vi "KeithleMatrixResistance.vi"() -> ()   [LabVIEW 2014]
uses:
  <vilib>/Utility/file.llb/Write To Spreadsheet File (DBL).vi
panel:
  out "Resistance":dbl
  out "Array":bool[][](array[boolean])
  in  "GPIB Address":string="12"
  out "String":string
  in  "Set values for testing contacts":bool
  out "Output Current (A)":dbl
  out "Output Voltage (V)":dbl
  out "Compliance limit (V)":dbl
  out "Current Range":u16(ring) items=["100 nA", "1 uA", "10 uA", "100 uA", "1 mA", "10 mA", "100 mA", "1 A"]
  out "Voltage Range":u16(ring) items=["200 mV", "2 V", "20 V", "200 V"]
  out "Current (sourse)":dbl
  out "Voltage (sourse)":dbl
  out "ComplianceIndicator":bool
  out "Compliance limit (A)":dbl
  out "Source Function":u16(ring)=1 items=["Current Source", "Voltage Source"]
  out "Sence Mode":u16(ring) items=["2-wire", "4-wire"]
  in  "ON/OFF channel":bool
  out "ON/OFF indicator":bool
  in  "error in (no error)":errorcluster
  out "error out":errorcluster
  # "Channel\nB"
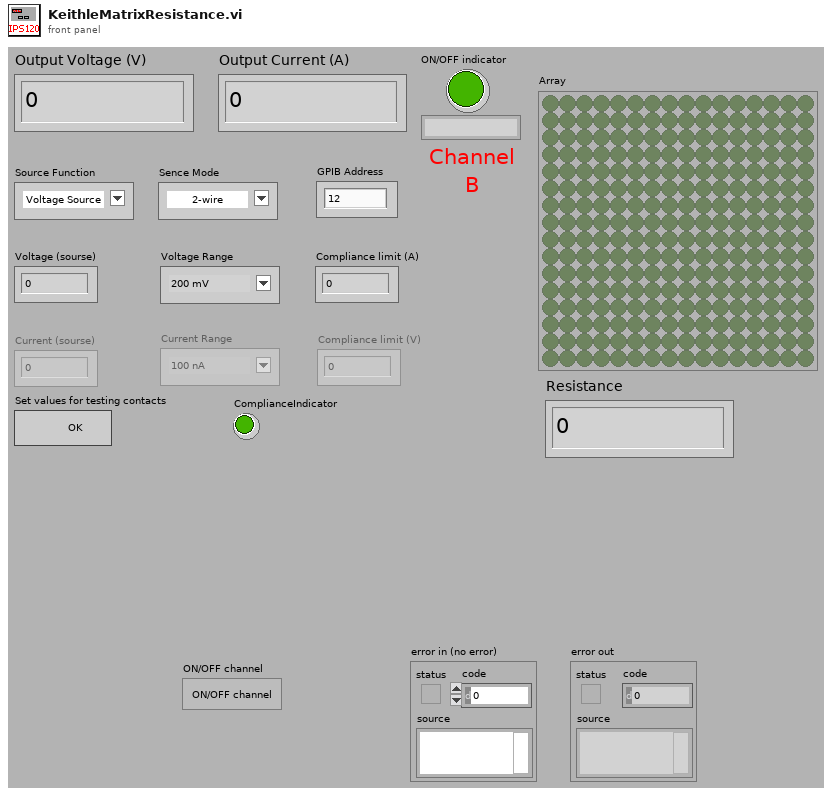
[diagram p1: front panel]
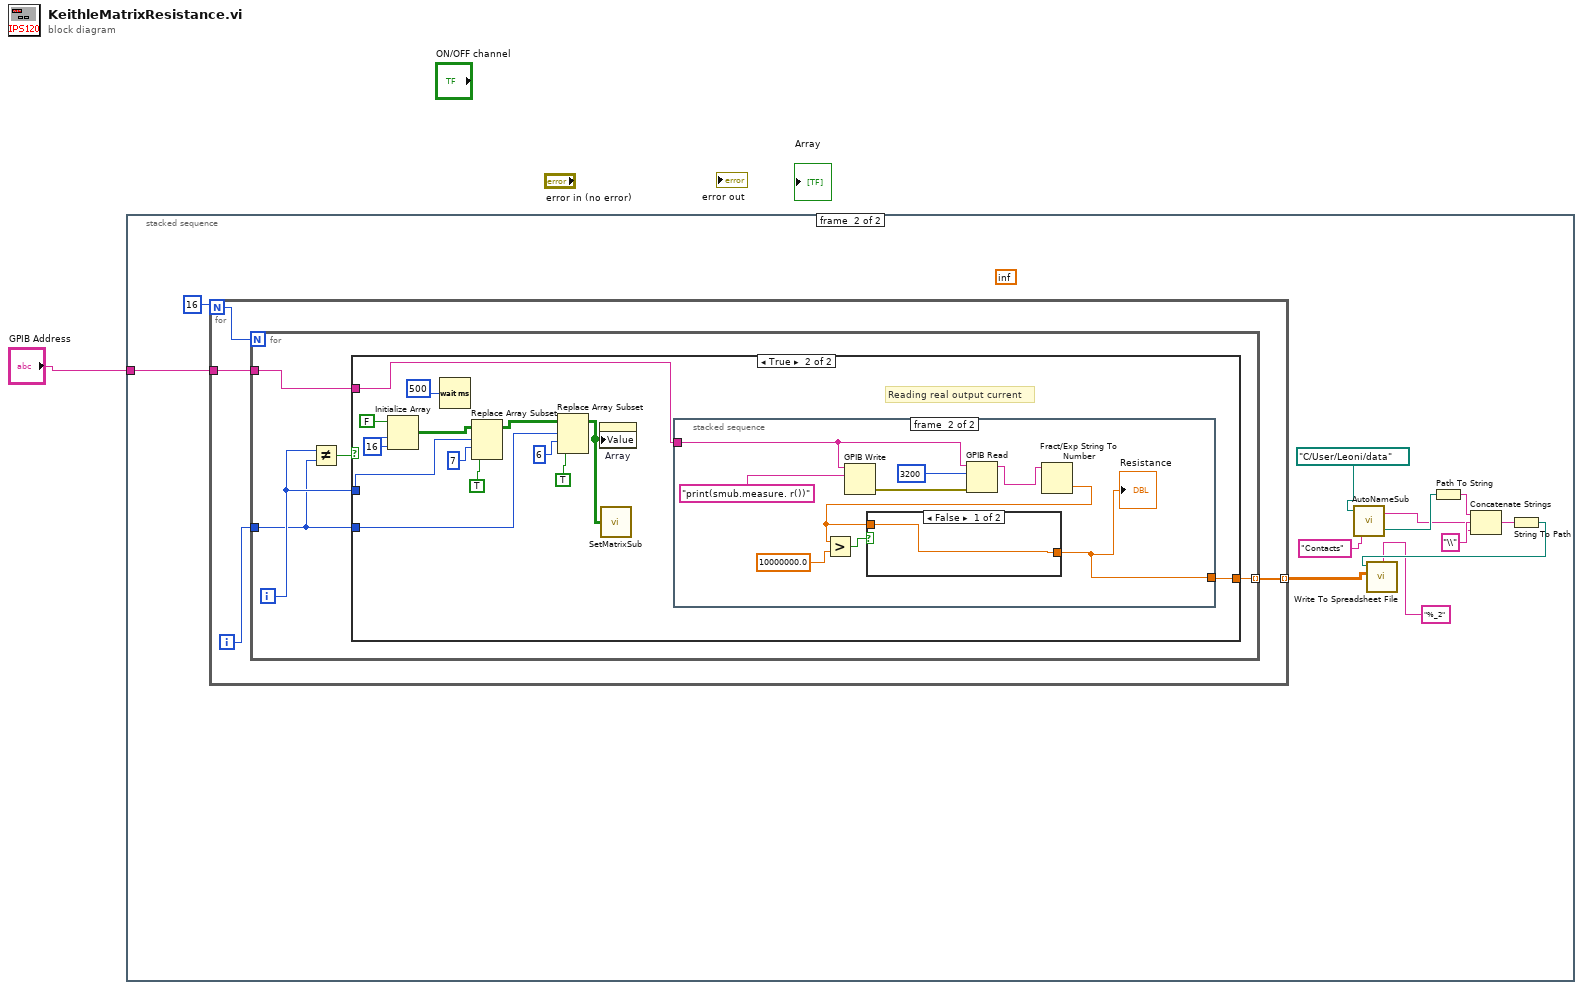
[diagram p0: block diagram]
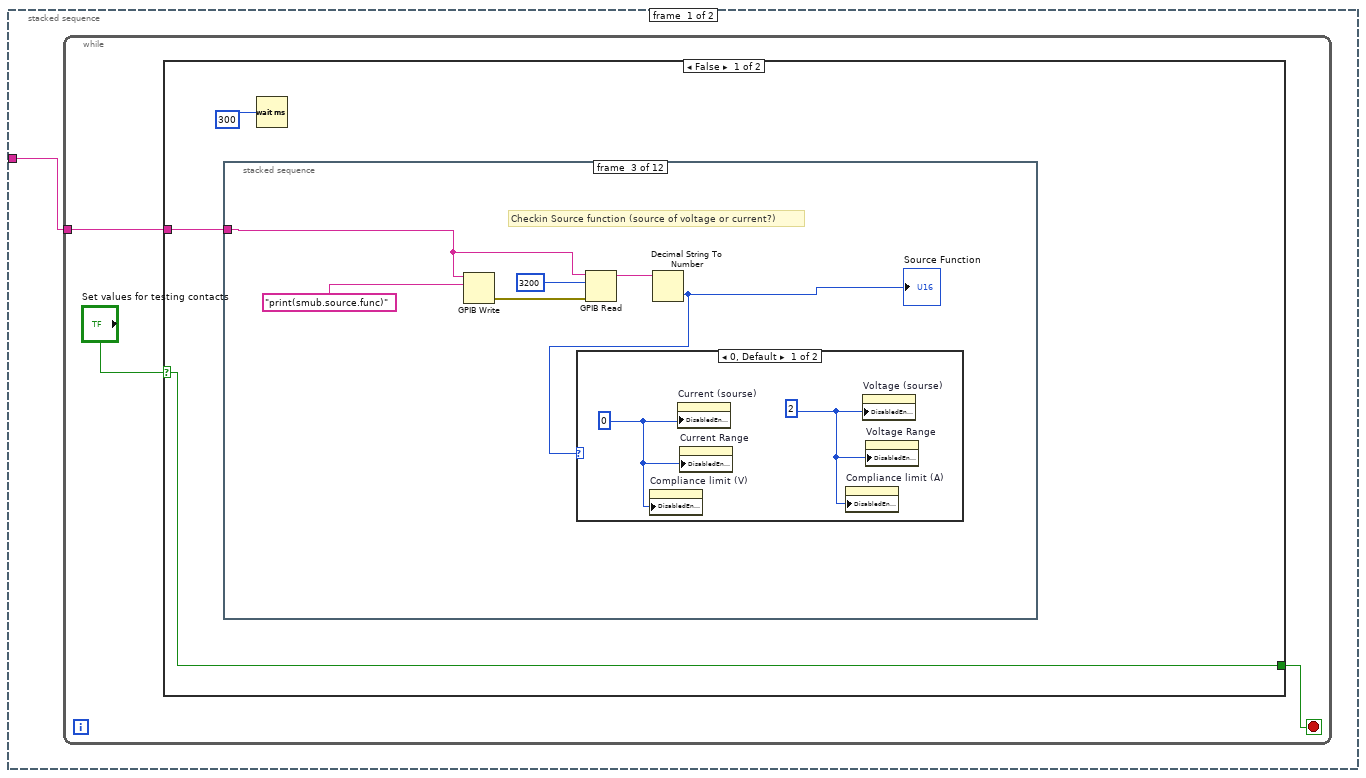
[diagram p2: hidden frame]
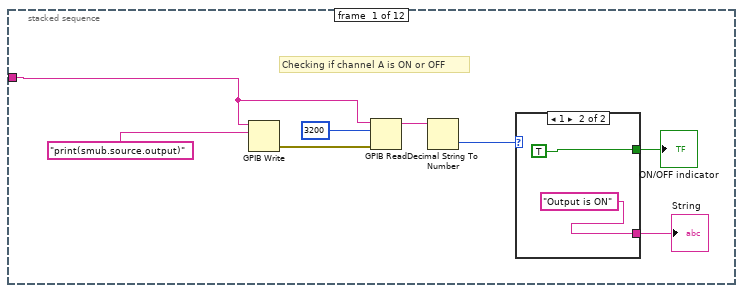
[diagram p3: hidden frame]
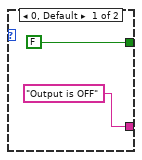
[diagram p4: hidden frame]
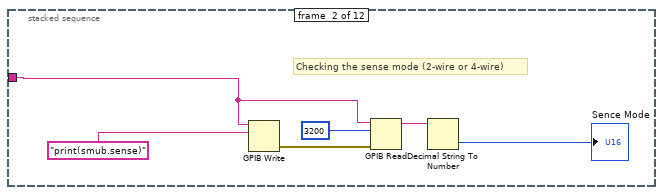
[diagram p5: hidden frame]
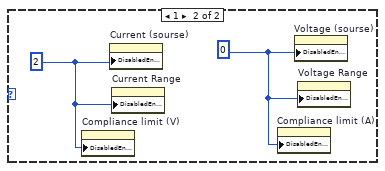
[diagram p6: hidden frame]
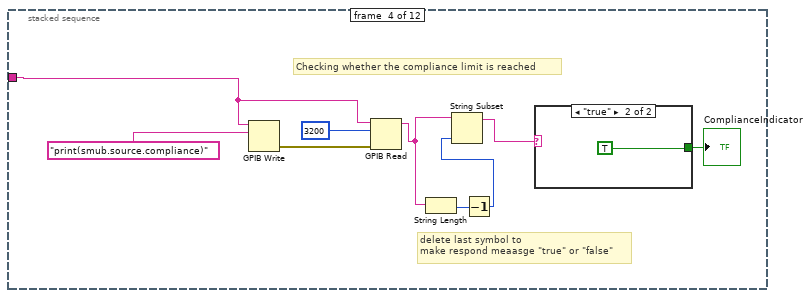
[diagram p7: hidden frame]
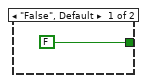
[diagram p8: hidden frame]
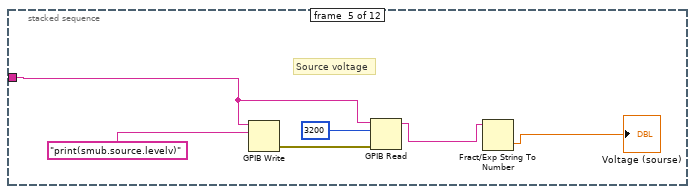
[diagram p9: hidden frame]
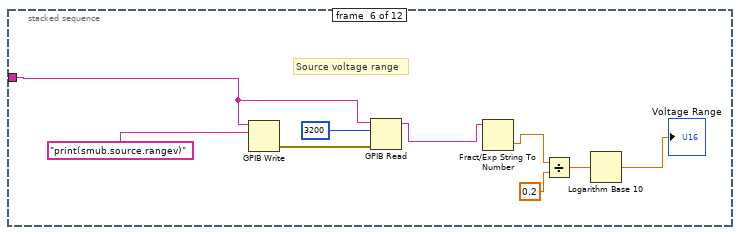
[diagram p10: hidden frame]
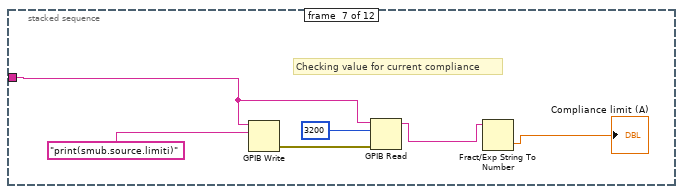
[diagram p11: hidden frame]
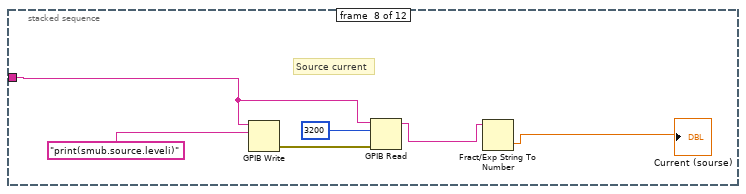
[diagram p12: hidden frame]
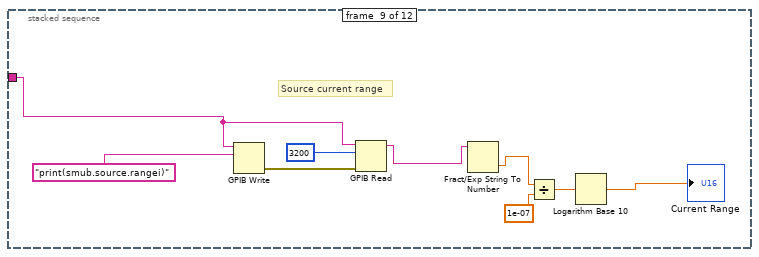
[diagram p13: hidden frame]
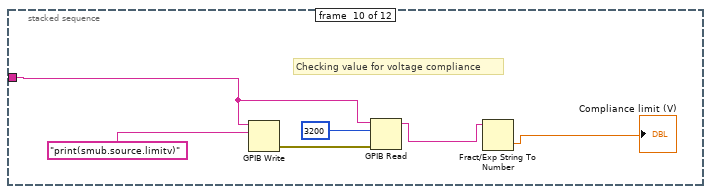
[diagram p14: hidden frame]
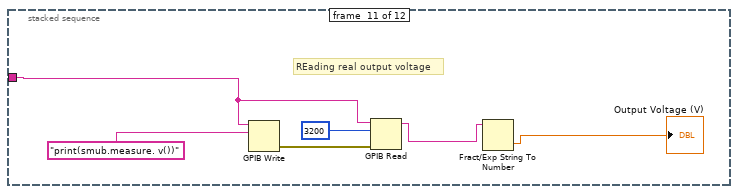
[diagram p15: hidden frame]
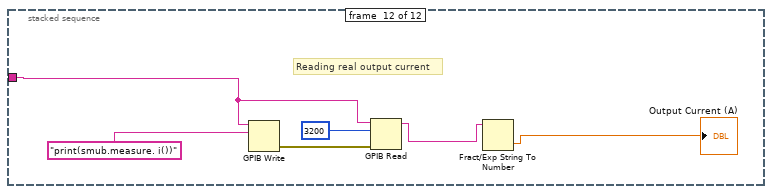
[diagram p16: hidden frame]
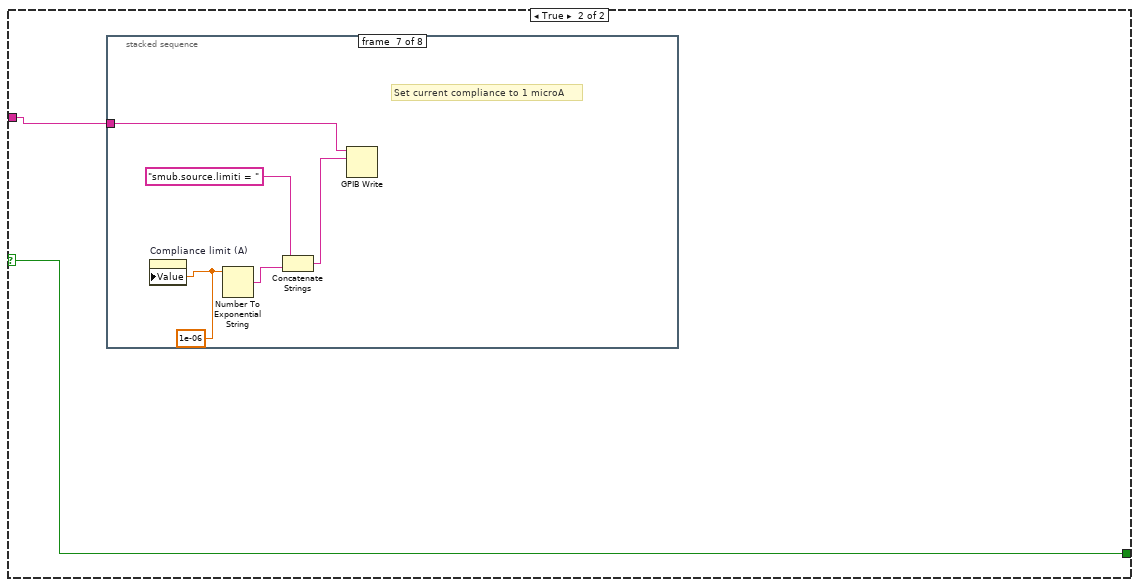
[diagram p17: hidden frame]
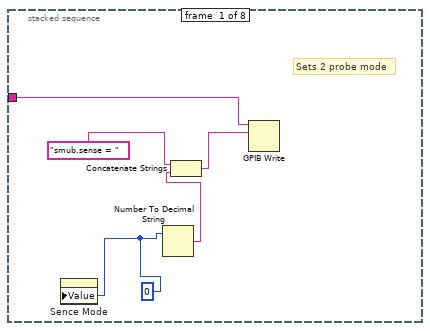
[diagram p18: hidden frame]
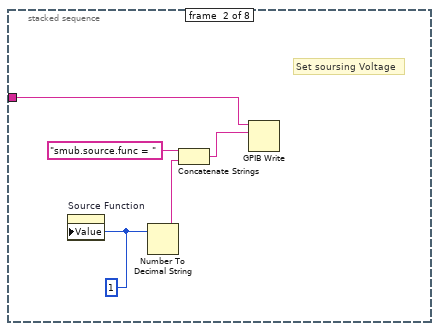
[diagram p19: hidden frame]
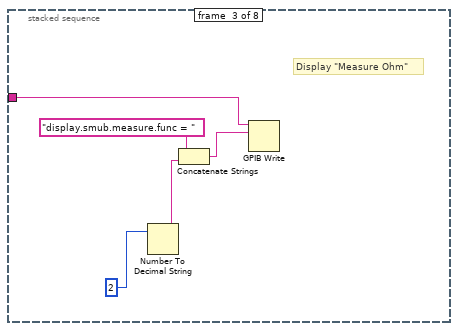
[diagram p20: hidden frame]
diagram:
  n1 = stacked-sequence {
    tunnel: "GPIB Address" -> [w2 w153]
    frame #0 {
      n2 = while {
        tunnel: w2 -> [w3]
        stop <- w4 stop-if-true
        n3 = case shown="False" "Set values for testing contacts" {
          selector: "Set values for testing contacts" -> [w7 w102]
          tunnel: w3 -> [w8 w103]
          tunnel: [w7 w102] -> w4
          frame False {
            n4 = stacked-sequence {
              tunnel: w8 -> [w9 w21 w27 w37 w48 w54 w63 w69 w75 w84 w90 w96]
              frame #0 {
                # "Checking if channel A is ON or OFF"
                n5 = GPIB Write(0:w9, 1:"print(smub.source.output)") -> (6:w16:errorcluster)  [unwired: 3 in, 1 out]
                n6 = GPIB Read(0:w9, 1:3200, 3:w16) -> (5:w13:string)  [unwired: 2 in, 2 out]
                n7 = Decimal String To Number(string=w13) -> (number=w12:i32)  [unwired: 2 in, 1 out]
                n8 = case shown="1" w12 {
                  tunnel: [FALSE TRUE] -> w11
                  tunnel: ["Output is OFF" "Output is ON"] -> w10
                  frame 0, Default {
                  }
                  frame 1 {
                  }
                }
                "ON/OFF indicator" <- w11
                "String" <- w10
              }
              frame #1 {
                # "Checking the sense mode (2-wire or 4-wire)"
                n9 = GPIB Write(0:w21, 1:"print(smub.sense)") -> (6:w26:errorcluster)  [unwired: 3 in, 1 out]
                n10 = GPIB Read(0:w21, 1:3200, 3:w26) -> (5:w23:string)  [unwired: 2 in, 2 out]
                n11 = Decimal String To Number(string=w23) -> (number=→"Sence Mode":i32)  [unwired: 2 in, 1 out]
              }
              frame #2 {
                # "Checkin Source function (source of voltage or current?)"
                n12 = GPIB Write(0:w27, 1:"print(smub.source.func)") -> (6:w32:errorcluster)  [unwired: 3 in, 1 out]
                n13 = GPIB Read(0:w27, 1:3200, 3:w32) -> (5:w29:string)  [unwired: 2 in, 2 out]
                n14 = Decimal String To Number(string=w29) -> (number=w28:i32)  [unwired: 2 in, 1 out]
                "Source Function" <- w28
                n15 = case shown="0, Default" w28 {
                  frame 0, Default {
                    w33 = 2
                    w34 = 0
                    n16 = property on="Compliance limit (V)" class="DigNum (strict)"("DisabledEnum"=w34) -> ()  [unwired: 2 in, 2 out]
                    n17 = property on="Current (sourse)" class="DigNum (strict)"("DisabledEnum"=w34) -> ()  [unwired: 2 in, 2 out]
                    n18 = property on="Current Range" class="Ring (strict)"("DisabledEnum"=w34) -> ()  [unwired: 2 in, 2 out]
                    n19 = property on="Compliance limit (A)" class="DigNum (strict)"("DisabledEnum"=w33) -> ()  [unwired: 2 in, 2 out]
                    n20 = property on="Voltage (sourse)" class="DigNum (strict)"("DisabledEnum"=w33) -> ()  [unwired: 2 in, 2 out]
                    n21 = property on="Voltage Range" class="Ring (strict)"("DisabledEnum"=w33) -> ()  [unwired: 2 in, 2 out]
                  }
                  frame 1 {
                    w35 = 0
                    w36 = 2
                    n22 = property on="Compliance limit (V)" class="DigNum (strict)"("DisabledEnum"=w36) -> ()  [unwired: 2 in, 2 out]
                    n23 = property on="Current (sourse)" class="DigNum (strict)"("DisabledEnum"=w36) -> ()  [unwired: 2 in, 2 out]
                    n24 = property on="Current Range" class="Ring (strict)"("DisabledEnum"=w36) -> ()  [unwired: 2 in, 2 out]
                    n25 = property on="Compliance limit (A)" class="DigNum (strict)"("DisabledEnum"=w35) -> ()  [unwired: 2 in, 2 out]
                    n26 = property on="Voltage (sourse)" class="DigNum (strict)"("DisabledEnum"=w35) -> ()  [unwired: 2 in, 2 out]
                    n27 = property on="Voltage Range" class="Ring (strict)"("DisabledEnum"=w35) -> ()  [unwired: 2 in, 2 out]
                  }
                }
              }
              frame #3 {
                # "delete last symbol to\nmake respond meaasge \"true\" or \"false\""
                # "Checking whether the compliance limit is reached"
                n28 = GPIB Write(0:w37, 1:"print(smub.source.compliance)") -> (6:w45:errorcluster)  [unwired: 3 in, 1 out]
                n29 = GPIB Read(0:w37, 1:3200, 3:w45) -> (5:w39:string)  [unwired: 2 in, 2 out]
                n30 = String Length(string=w39) -> (length=w41:i32)
                n31 = Decrement(x=w41) -> (x-1=w40:i32)
                n32 = String Subset(string=w39, length (rest)=w40) -> (substring=w38:string)  [unwired: 1 in]
                n33 = case shown="\"true\"" w38 {
                  tunnel: [FALSE TRUE] -> w42
                  frame "False", Default {
                  }
                  frame "true" {
                  }
                }
                "ComplianceIndicator" <- w42
              }
              frame #4 {
                # "Source voltage"
                n34 = GPIB Write(0:w48, 1:"print(smub.source.levelv)") -> (6:w53:errorcluster)  [unwired: 3 in, 1 out]
                n35 = GPIB Read(0:w48, 1:3200, 3:w53) -> (5:w50:string)  [unwired: 2 in, 2 out]
                n36 = Fract/Exp String To Number(string=w50) -> (number=→"Voltage (sourse)":dbl)  [unwired: 3 in, 1 out]
              }
              frame #5 {
                # "Source voltage range"
                n37 = GPIB Write(0:w54, 1:"print(smub.source.rangev)") -> (6:w62:errorcluster)  [unwired: 3 in, 1 out]
                n38 = GPIB Read(0:w54, 1:3200, 3:w62) -> (5:w59:string)  [unwired: 2 in, 2 out]
                n39 = Fract/Exp String To Number(string=w59) -> (number=w57:dbl)  [unwired: 3 in, 1 out]
                n40 = Divide(x=w57, y=0.2) -> (x/y=w56:dbl)
                n41 = Logarithm Base 10(1:w56) -> (0:→"Voltage Range":dbl)
              }
              frame #6 {
                # "Checking value for current compliance"
                n42 = GPIB Write(0:w63, 1:"print(smub.source.limiti)") -> (6:w68:errorcluster)  [unwired: 3 in, 1 out]
                n43 = GPIB Read(0:w63, 1:3200, 3:w68) -> (5:w65:string)  [unwired: 2 in, 2 out]
                n44 = Fract/Exp String To Number(string=w65) -> (number=→"Compliance limit (A)":dbl)  [unwired: 3 in, 1 out]
              }
              frame #7 {
                # "Source current"
                n45 = GPIB Write(0:w69, 1:"print(smub.source.leveli)") -> (6:w74:errorcluster)  [unwired: 3 in, 1 out]
                n46 = GPIB Read(0:w69, 1:3200, 3:w74) -> (5:w71:string)  [unwired: 2 in, 2 out]
                n47 = Fract/Exp String To Number(string=w71) -> (number=→"Current (sourse)":dbl)  [unwired: 3 in, 1 out]
              }
              frame #8 {
                # "Source current range"
                n48 = GPIB Write(0:w75, 1:"print(smub.source.rangei)") -> (6:w83:errorcluster)  [unwired: 3 in, 1 out]
                n49 = GPIB Read(0:w75, 1:3200, 3:w83) -> (5:w80:string)  [unwired: 2 in, 2 out]
                n50 = Fract/Exp String To Number(string=w80) -> (number=w78:dbl)  [unwired: 3 in, 1 out]
                n51 = Divide(x=w78, y=1e-07) -> (x/y=w77:dbl)
                n52 = Logarithm Base 10(1:w77) -> (0:→"Current Range":dbl)
              }
              frame #9 {
                # "Checking value for voltage compliance"
                n53 = GPIB Write(0:w84, 1:"print(smub.source.limitv)") -> (6:w89:errorcluster)  [unwired: 3 in, 1 out]
                n54 = GPIB Read(0:w84, 1:3200, 3:w89) -> (5:w86:string)  [unwired: 2 in, 2 out]
                n55 = Fract/Exp String To Number(string=w86) -> (number=→"Compliance limit (V)":dbl)  [unwired: 3 in, 1 out]
              }
              frame #10 {
                # "REading real output voltage"
                n56 = GPIB Write(0:w90, 1:"print(smub.measure. v())") -> (6:w95:errorcluster)  [unwired: 3 in, 1 out]
                n57 = GPIB Read(0:w90, 1:3200, 3:w95) -> (5:w92:string)  [unwired: 2 in, 2 out]
                n58 = Fract/Exp String To Number(string=w92) -> (number=→"Output Voltage (V)":dbl)  [unwired: 3 in, 1 out]
              }
              frame #11 {
                # "Reading real output current"
                n59 = GPIB Write(0:w96, 1:"print(smub.measure. i())") -> (6:w101:errorcluster)  [unwired: 3 in, 1 out]
                n60 = GPIB Read(0:w96, 1:3200, 3:w101) -> (5:w98:string)  [unwired: 2 in, 2 out]
                n61 = Fract/Exp String To Number(string=w98) -> (number=→"Output Current (A)":dbl)  [unwired: 3 in, 1 out]
              }
            }
            n62 = Wait (ms)(milliseconds to wait=300) -> ()  [unwired: 1 out]
          }
          frame True {
            n63 = stacked-sequence {
              tunnel: w103 -> [w105 w110 w115 _ w120 w125 w133 w138]
              frame #0 {
                w104 = 0
                # "Sets 2 probe mode"
                n64 = property on="Sence Mode" class="Ring (strict)"("Value"=w104) -> ()  [unwired: 2 in, 2 out]
                n65 = Number To Decimal String(number=w104) -> (decimal integer string=w107:string)  [unwired: 1 in]
                n66 = Concatenate Strings("smub.sense = ", w107) -> (w106:string)
                n67 = GPIB Write(0:w105, 1:w106) -> ()  [unwired: 3 in, 2 out]
              }
              frame #1 {
                w109 = 1
                # "Set soursing Voltage"
                n68 = property on="Source Function" class="Ring (strict)"("Value"=w109) -> ()  [unwired: 2 in, 2 out]
                n69 = Number To Decimal String(number=w109) -> (decimal integer string=w112:string)  [unwired: 1 in]
                n70 = Concatenate Strings("smub.source.func = ", w112) -> (w111:string)
                n71 = GPIB Write(0:w110, 1:w111) -> ()  [unwired: 3 in, 2 out]
              }
              frame #2 {
                # "Display \"Measure Ohm\""
                n72 = Number To Decimal String(number=2) -> (decimal integer string=w117:string)  [unwired: 1 in]
                n73 = Concatenate Strings("display.smub.measure.func = ", w117) -> (w116:string)
                n74 = GPIB Write(0:w115, 1:w116) -> ()  [unwired: 3 in, 2 out]
              }
              frame #3 {
              }
              frame #4 {
                w119 = 0.01
                # "Set Output voltage to 10 mV"
                n75 = property on="Voltage (sourse)" class="DigNum (strict)"("Value"=w119) -> ()  [unwired: 2 in, 2 out]
                n76 = Number To Exponential String(number=w119) -> (E-format string=w122:string)  [unwired: 3 in]
                n77 = Concatenate Strings("smub.source.levelv = ", w122) -> (w121:string)
                n78 = GPIB Write(0:w120, 1:w121) -> ()  [unwired: 3 in, 2 out]
              }
              frame #5 {
                w124 = 0
                # "Set to lowest voltage range (200 mV)"
                n79 = property on="Voltage Range" class="Ring (strict)"("Value"=w124) -> ()  [unwired: 2 in, 2 out]
                n80 = Power Of 10(x=w124) -> (10^x=w127:dbl)
                n81 = Multiply(x=w127, y=0.2) -> (x*y=w126:dbl)
                n82 = Number To Exponential String(number=w126) -> (E-format string=w131:string)  [unwired: 3 in]
                n83 = Concatenate Strings("smub.source.rangev = ", w131) -> (w129:string)
                n84 = GPIB Write(0:w125, 1:w129) -> ()  [unwired: 3 in, 2 out]
              }
              frame #6 {
                w132 = 1e-06
                # "Set current compliance to 1 microA"
                n85 = property on="Compliance limit (A)" class="DigNum (strict)"("Value"=w132) -> ()  [unwired: 2 in, 2 out]
                n86 = Number To Exponential String(number=w132) -> (E-format string=w136:string)  [unwired: 3 in]
                n87 = Concatenate Strings("smub.source.limiti = ", w136) -> (w134:string)
                n88 = GPIB Write(0:w133, 1:w134) -> ()  [unwired: 3 in, 2 out]
              }
              frame #7 {
                w137 = TRUE
                # "Turn ON channel B"
                n89 = property on="ON/OFF indicator" class="Bool (strict)"("Value"=w137) -> ()  [unwired: 2 in, 2 out]
                n90 = Boolean To (0,1)(Boolean=w137) -> (0, 1=w142:i16)
                n91 = Number To Decimal String(number=w142) -> (decimal integer string=w140:string)  [unwired: 1 in]
                n92 = Concatenate Strings("smub.source.output = ", w140) -> (w139:string)
                n93 = GPIB Write(0:w138, 1:w139) -> ()  [unwired: 3 in, 2 out]
              }
            }
          }
        }
      }
    }
    frame #1 {
      (unwired) inf
      n94 = for {
        N: 16 -> [w157]
        tunnel: w153 -> [w156]
        tunnel: [w155] -> w152 mode=indexing
        i -> [w158]
        n95 = for {
          N: w157 -> [_]
          tunnel: w158 -> [w161]
          tunnel: w156 -> [w160]
          tunnel: [w159] -> w155 mode=indexing
          i -> [w162]
          n96 = Not Equal?(x=w162, y=w161) -> (x != y?=w163:bool)
          n97 = case shown="True" w163 {
            tunnel: w162 -> [_ w174]
            tunnel: w161 -> [_ w170]
            tunnel: w160 -> [_ w166]
            tunnel: [0.0 w165] -> w159
            frame False {
            }
            frame True {
              w177 = 16
              # "Reading real output current"
              n98 = Initialize Array(FALSE, w177, w177) -> (w176:bool[][])
              n99 = Wait (ms)(milliseconds to wait=500) -> ()  [unwired: 1 out]
              n100 = Replace Array Subset(array=w176, new element=TRUE, index (row)=w174, index (col)=7) -> (w169:bool[][])
              n101 = Replace Array Subset(array=w169, new element=TRUE, index (row)=w170, index (col)=6) -> (w167:bool[][])
              n102 = property on="Array" class="Arr (strict)"("Value"=w167) -> ()  [unwired: 2 in, 2 out]
              n103 = call "SetMatrixSub.vi"("Array"=w167) -> ()  [unwired: 1 in]
              n104 = stacked-sequence {
                tunnel: w166 -> [_ w184]
                tunnel: [_ w180] -> w165
                frame #0 {
                  n105 = Wait (ms)(milliseconds to wait=500) -> ()  [unwired: 1 out]
                }
                frame #1 {
                  n106 = GPIB Write(0:w184, 1:"print(smub.measure. r())") -> (6:w185:errorcluster)  [unwired: 3 in, 1 out]
                  n107 = GPIB Read(0:w184, 1:3200, 3:w185) -> (5:w188:string)  [unwired: 2 in, 2 out]
                  n108 = Fract/Exp String To Number(string=w188) -> (number=w181:dbl)  [unwired: 3 in, 1 out]
                  n109 = Greater?(x=w181, y=10000000.0) -> (0:w183:bool)
                  n110 = case shown="False" w183 {
                    tunnel: [w189 inf] -> w180
                    tunnel: w181 -> [w189 _]
                    frame False {
                    }
                    frame True {
                    }
                  }
                  "Resistance" <- w180
                }
              }
            }
          }
        }
      }
      n111 = call "AutoNameSub.vi"("Custom Folder"="Contacts", "User Data Folder"=path "C:/User/Leoni/data") -> ("created path"=w147:path, "String"=w146:string)  [unwired: 1 in]
      n112 = Path To String(path=w147) -> (string=w148:string)
      n113 = Concatenate Strings(w148, "\\", w146) -> (w150:string)
      n114 = String To Path(string=w150) -> (path=w145:path)
      n115 = call-poly <vilib>:"Write To Spreadsheet File.vi"("format (%.3f)"="%_2", "2D data"=w152, "file path (dialog if empty)"=w145) -> ()  [unwired: 5 in, 1 out]
    }
  }
